vi "TL_ALL_on_v2.vi"(8 "error in":errorcluster, 10 "Settings":T2={"Module"=enum."On Line LD", "OnLineTEC"=19.473, "OnLineLD"=0.155, "OffLineTEC"=18.541, "OffLineLD"=0.155, "EtalonTEC"=28.1, "TSOA-TEC"=20.0007572} {"OffLineLD" min=0.0 max=0.17 step=0.001 format="%.3p"; "OnLineLD" min=0.0 max=0.17 step=0.001 format="%.3p"; "TSOA-TEC" format="%.2g"; "EtalonTEC" format="%.2g"; "OffLineTEC" min=16.0 max=28.0 step=0.1 format="%.3g"; "OnLineTEC" min=16.0 max=28.0 step=0.1 format="%.3g"}, 11 "Device In":refnum<visa-resource-name>="ThorLabs") -> ()   [LabVIEW 2012]
panel:
  out "Readings":T1={"OnLineTEC"=19.6115971, "OnLineLD"=0.00013867188, "OffLineTEC"=18.6689701, "OffLineLD"=0.0, "EtalonTEC"=22.7138939, "TSOA-TEC"=22.3323307, "Pro8000"=TRUE, "OnLine TEC"=TRUE, "OnLine LD"=TRUE, "OffLine TEC"=TRUE, "OffLine LD"=TRUE, "Etalon TEC"=TRUE, "TSOA TEC"=TRUE} {"OffLineLD" format="%.3p"; "OnLineLD" format="%.3p"; "TSOA-TEC" format="%.3g"; "EtalonTEC" format="%.3g"; "OffLineTEC" format="%.3g"; "OnLineTEC" format="%.3g"}
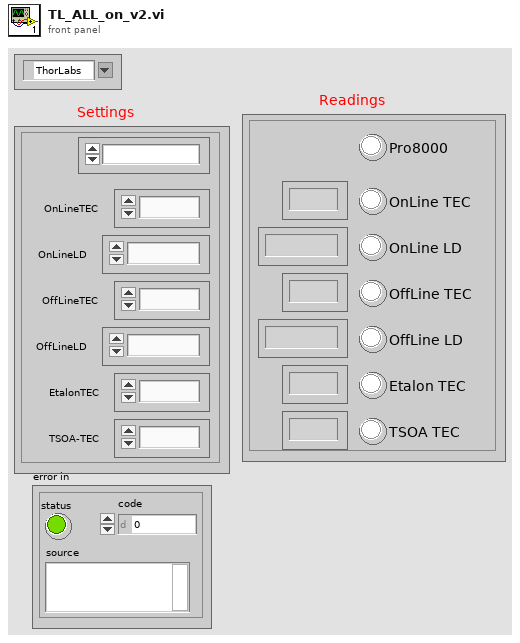
[diagram p1: front panel]
types:
  T1 = cluster{"OnLineTEC":dbl, "OnLineLD":dbl, "OffLineTEC":dbl, "OffLineLD":dbl, "EtalonTEC":dbl, "TSOA-TEC":dbl, "Pro8000":bool, "OnLine TEC":bool, "OnLine LD":bool, "OffLine TEC":bool, "OffLine LD":bool, "Etalon TEC":bool, "TSOA TEC":bool}
  T2 = cluster{"Module":enum16{"On Line TEC", "On Line LD", "Off Line TEC", "Off Line LD", "Etalon TEC", "TSOA TEC"}, "OnLineTEC":dbl, "OnLineLD":dbl, "OffLineTEC":dbl, "OffLineLD":dbl, "EtalonTEC":dbl, "TSOA-TEC":dbl}
  T3 = enum16{"Open_TL", "Close_TL", "Verify_ID", "TEC_Sensor", "SET", "READ", "ON", "OFF", "Set_Limits", "Read_Limits", "Enable_Status", "Read_Status"}
  T4 = enum16{"On Line TEC", "On Line LD", "Off Line TEC", "Off Line LD", "Etalon TEC", "TSOA TEC"}
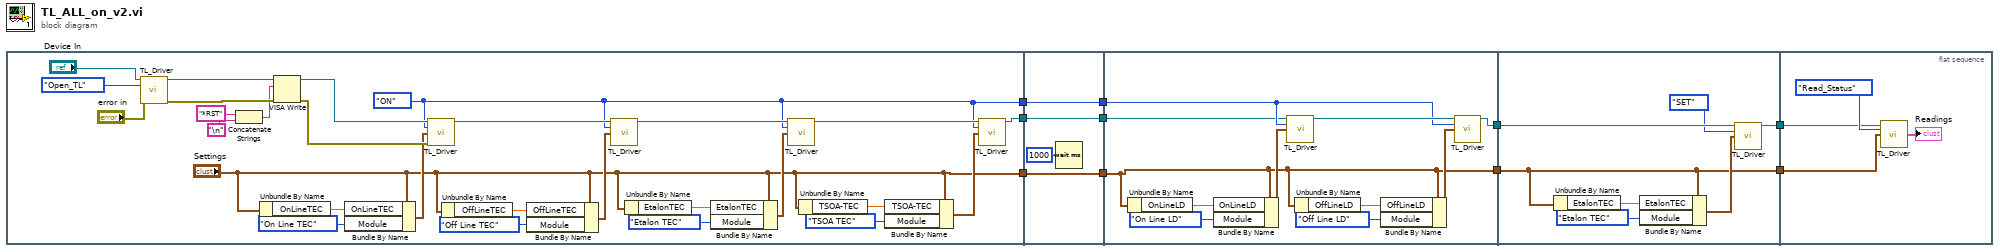
[diagram p0: block diagram]
diagram:
  n1 = flat-sequence {
    tunnel: [w14] -> w9
    tunnel: [w13] -> w7
    tunnel: ["Settings"] -> w5
    tunnel: [w42] -> w10
    tunnel: w9 -> [w42]
    tunnel: [w41] -> w8
    tunnel: w7 -> [w41]
    tunnel: [w40] -> w6
    tunnel: w5 -> [w40]
    tunnel: w10 -> [w46]
    tunnel: w8 -> [w45]
    tunnel: w6 -> [w43]
    tunnel: [w44] -> w4
    tunnel: [w43] -> w2
    tunnel: w4 -> [w58]
    tunnel: [w57] -> w3
    tunnel: w2 -> [w54]
    tunnel: [w54] -> w1
    tunnel: w3 -> [w62]
    tunnel: w1 -> [w61]
    frame #0 {
      w14 = T3."ON" ("Commands")
      n2 = call "TL_Driver.vi"("Device In"="Device In", "Commands"=T3."Open_TL", "error in"="error in") -> ("Device Out"=w34:refnum<visa-resource-name>, "error out"=w33:errorcluster)  [unwired: 9 in, 2 out]
      n3 = Concatenate Strings("*RST" ("string"), "\n") -> (w32:string)
      n4 = Unbundle By Name("Settings") -> ("OnLineTEC"=w19:dbl)
      n5 = VISA Write(VISA resource name=w34, write buffer=w32, error in (no error)=w33) -> (VISA resource name out=w35:refnum<visa-resource-name>, error out=w36:errorcluster)  [unwired: 1 out]
      n6 = Bundle By Name(cluster="Settings", "OnLineTEC"=w19, "Module"=T4."On Line TEC") -> (w21:T2)
      n7 = call "TL_Driver.vi"("Device In"=w35, "Commands"=w14, "Settings"=w21, "error in"=w36) -> ("Device Out"=w17:refnum<visa-resource-name>)  [unwired: 8 in, 3 out]
      n8 = Unbundle By Name("Settings") -> ("OffLineTEC"=w22:dbl)
      n9 = Bundle By Name(cluster="Settings", "OffLineTEC"=w22, "Module"=T4."Off Line TEC") -> (w24:T2)
      n10 = call "TL_Driver.vi"("Device In"=w17, "Commands"=w14, "Settings"=w24) -> ("Device Out"=w18:refnum<visa-resource-name>)  [unwired: 9 in, 3 out]
      n11 = Unbundle By Name("Settings") -> ("EtalonTEC"=w25:dbl)
      n12 = Bundle By Name(cluster="Settings", "EtalonTEC"=w25, "Module"=T4."Etalon TEC") -> (w27:T2)
      n13 = call "TL_Driver.vi"("Device In"=w18, "Commands"=w14, "Settings"=w27) -> ("Device Out"=w16:refnum<visa-resource-name>)  [unwired: 9 in, 3 out]
      n14 = Unbundle By Name("Settings") -> ("TSOA-TEC"=w28:dbl)
      n15 = Bundle By Name(cluster="Settings", "TSOA-TEC"=w28, "Module"=T4."TSOA TEC") -> (w15:T2)
      n16 = call "TL_Driver.vi"("Device In"=w16, "Commands"=w14, "Settings"=w15) -> ("Device Out"=w13:refnum<visa-resource-name>)  [unwired: 9 in, 3 out]
    }
    frame #1 {
      n17 = Wait (ms)(milliseconds to wait=u32 1000) -> ()  [unwired: 1 out]
    }
    frame #2 {
      n18 = Unbundle By Name(w43) -> ("OnLineLD"=w47:dbl)
      n19 = Bundle By Name(cluster=w43, "OnLineLD"=w47, "Module"=T4."On Line LD") -> (w49:T2)
      n20 = call "TL_Driver.vi"("Device In"=w45, "Commands"=w46, "Settings"=w49) -> ("Device Out"=w52:refnum<visa-resource-name>)  [unwired: 9 in, 3 out]
      n21 = Unbundle By Name(w43) -> ("OffLineLD"=w50:dbl)
      n22 = Bundle By Name(cluster=w43, "OffLineLD"=w50, "Module"=T4."Off Line LD") -> (w53:T2)
      n23 = call "TL_Driver.vi"("Device In"=w52, "Commands"=w46, "Settings"=w53) -> ("Device Out"=w44:refnum<visa-resource-name>)  [unwired: 9 in, 3 out]
    }
    frame #3 {
      n24 = Unbundle By Name(w54) -> ("EtalonTEC"=w59:dbl)
      n25 = Bundle By Name(cluster=w54, "EtalonTEC"=w59, "Module"=T4."Etalon TEC") -> (w55:T2)
      n26 = call "TL_Driver.vi"("Device In"=w58, "Commands"=T3."SET", "Settings"=w55) -> ("Device Out"=w57:refnum<visa-resource-name>)  [unwired: 9 in, 3 out]
    }
    frame #4 {
      n27 = call "TL_Driver.vi"("Device In"=w62, "Commands"=T3."Read_Status", "Settings"=w61) -> ("Readings"=→"Readings":T1)  [unwired: 9 in, 3 out]
    }
  }
